vi "hCreate Data Filename.vi"(8 "File number":i32, 9 "Combo Box":string(combo), 10 "File name":string, 11 "base path":path) -> (0 "error out":errorcluster, 3 "refnum out":refnum<file>)   [LabVIEW 2012]
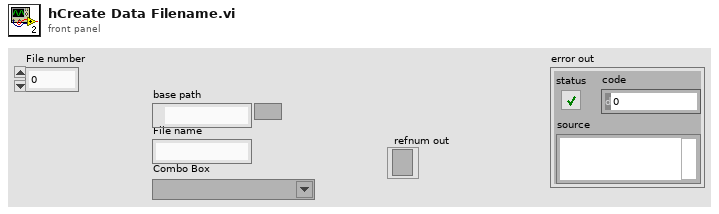
[diagram p1: front panel]
types:
  T1 = enum16{"open", "replace", "create", "open or create", "replace or create", "replace or create with confirmation"}
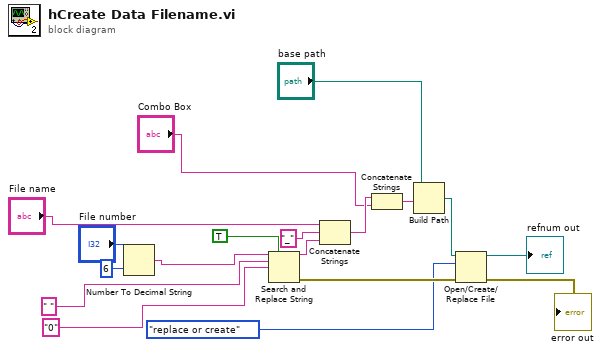
[diagram p0: block diagram]
diagram:
  n1 = Number To Decimal String(number="File number", width (-)=i16 6) -> (decimal integer string=w3:string)
  n2 = Search and Replace String(replace all?=TRUE ("replace all? (F)"), input string=w3, search string=" ", replace string="0" ("replace string (\"\")")) -> (result string=w14:string, error out=w16:errorcluster)  [unwired: 4 in, 2 out]
  n3 = Concatenate Strings("File name", "_" ("string"), w14) -> (w12:string)
  n4 = Concatenate Strings(w12, "Combo Box") -> (w15:string)
  n5 = Build Path(base path="base path", name or relative path=w15) -> (appended path=w17:path)
  n6 = Open/Create/Replace File(file path (use dialog)=w17, error in=w16, operation (0:open)=T1."replace or create") -> (refnum out=→"refnum out":refnum<file>, error out=→"error out":errorcluster)  [unwired: 3 in, 1 out]
